vi "migrate files.vi"() -> ()   [LabVIEW 2013]
uses:
  <vilib>/NI/Configuration Framework/class discovery singleton/class discovery singleton methods.ctl
  <vilib>/NI/Configuration Framework/tree serializer/memory hierarchy.ctl
  <vilib>/NI/Configuration Framework/tree serializer/full hierarchy.ctl
  <vilib>/NI/Configuration Framework/tree serializer/hierarchy element.ctl
  <vilib>/NI/Configuration Framework/serializable configuration/NISE_CEF_serializable configuration.lvclass
  <vilib>/NI/Tag Bus Data Framework/Configuration Editor/Classes/Systems/Systems.lvclass
  <vilib>/NI/Configuration Framework/serializable configuration/NISE_CEF_serializable configuration.lvclass/NISE_CEF_serializable configuration.ctl
  <vilib>/NI/Tag Bus Data Framework/core targets/cRIO/PLTarget cRIO.lvclass
  <vilib>/NI/Tag Bus Data Framework/core targets/PC/PLTarget PC.lvclass
  <vilib>/NI/TBM Engines/Standard Engine/Editor Node/Standard Engine Editor Node.lvclass
  <vilib>/NI/Configuration Framework/serializable node/NISE_CEF_serializable node.lvclass
  <vilib>/NI/Tag Bus Data Framework/Framework Configuration Classes/platypus configuration/PLConfigurationSerializer.lvlib
  <vilib>/NI/Configuration Framework/class discovery singleton/class discovery singleton.lvlib
  <vilib>/NI/Configuration Framework/tree serializer/NISE_CEF_TreeSerializer.lvlib
panel:
  out "created paths":path[](array[path])
  in  "cRIO (F=PC)":bool=TRUE
  in  "Path":path
  in  "Plugin Search Paths":path[](array[path])=[path "C:/Program Files (x86)/National Instruments/LabVIEW 2013/vi.lib/NI/Tag Bus Data Framework", path "C:/Program Files (x86)/National Instruments/LabVIEW 2013/vi.lib/NI/TBM Engines", path "C:/Program Files (x86)/National Instruments/LabVIEW 2013/vi.lib/NI/TBM Modules"]
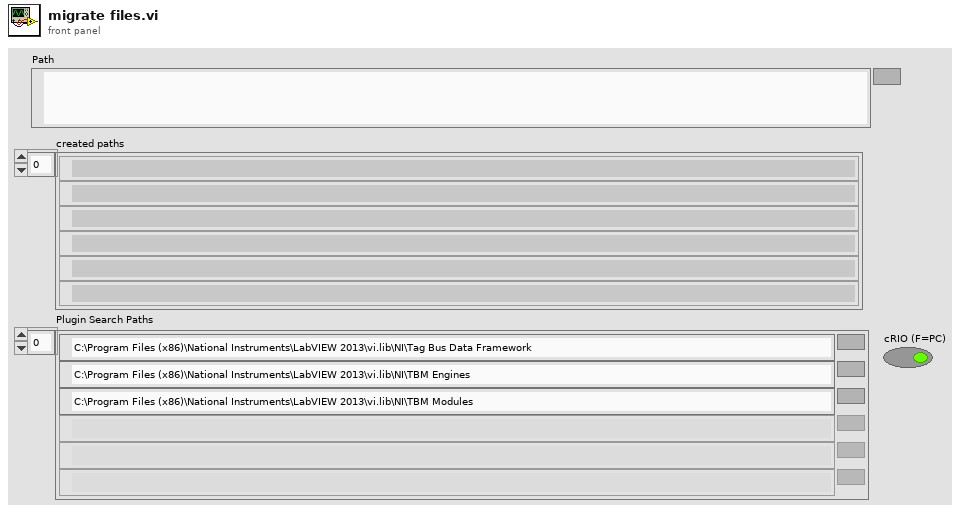
[diagram p1: front panel]
types:
  T1 = typedef "class discovery singleton.lvlib/class discovery singleton methods.ctl" = enum16{"add search paths", "load class by name", "list available classes", "get class path"}
  T2 = typedef "NISE_CEF_TreeSerializer.lvlib/memory hierarchy.ctl" = cluster{"hierarchy structure":T3, "instance data":refnum<class "NISE_CEF_serializable configuration.lvclass">[]}
  T3 = typedef "NISE_CEF_TreeSerializer.lvlib/full hierarchy.ctl" = cluster{"root":string, "hierarchy":T4[]}
  T4 = typedef "NISE_CEF_TreeSerializer.lvlib/hierarchy element.ctl" = cluster{"current node":string, "children":string[]}
  T5 = typedef "PLConfigurationSerializer.lvlib/systems cluster.ctl" = cluster{"System Configuration":refnum<class "PL_System Configuration.lvclass">, "targets":T6[]}
  T6 = typedef "PLConfigurationSerializer.lvlib/targets cluster.ctl" = cluster{"Target Configuration":refnum<class "PL_Target Configuration.lvclass">, "engines":T7[]}
  T7 = typedef "PLConfigurationSerializer.lvlib/engines cluster.ctl" = cluster{"engine configuration":refnum<class "engine configuration.lvclass">, "modules":refnum<class "TBM module configuration.lvclass">[]}
  T8 = typedef "NISE_CEF_TreeSerializer.lvlib/flat hierarchy.ctl" = cluster{"hierarchy structure":T3, "instance data":T9[]}
  T9 = typedef "NISE_CEF_TreeSerializer.lvlib/instance data.ctl" = cluster{"ID":string, "Alias":string, "class":string, "version":string, "data":string}
  T10 = typedef "NISE_CEF_TreeSerializer.lvlib/base file format.ctl" = cluster{"version":string, "data":string}
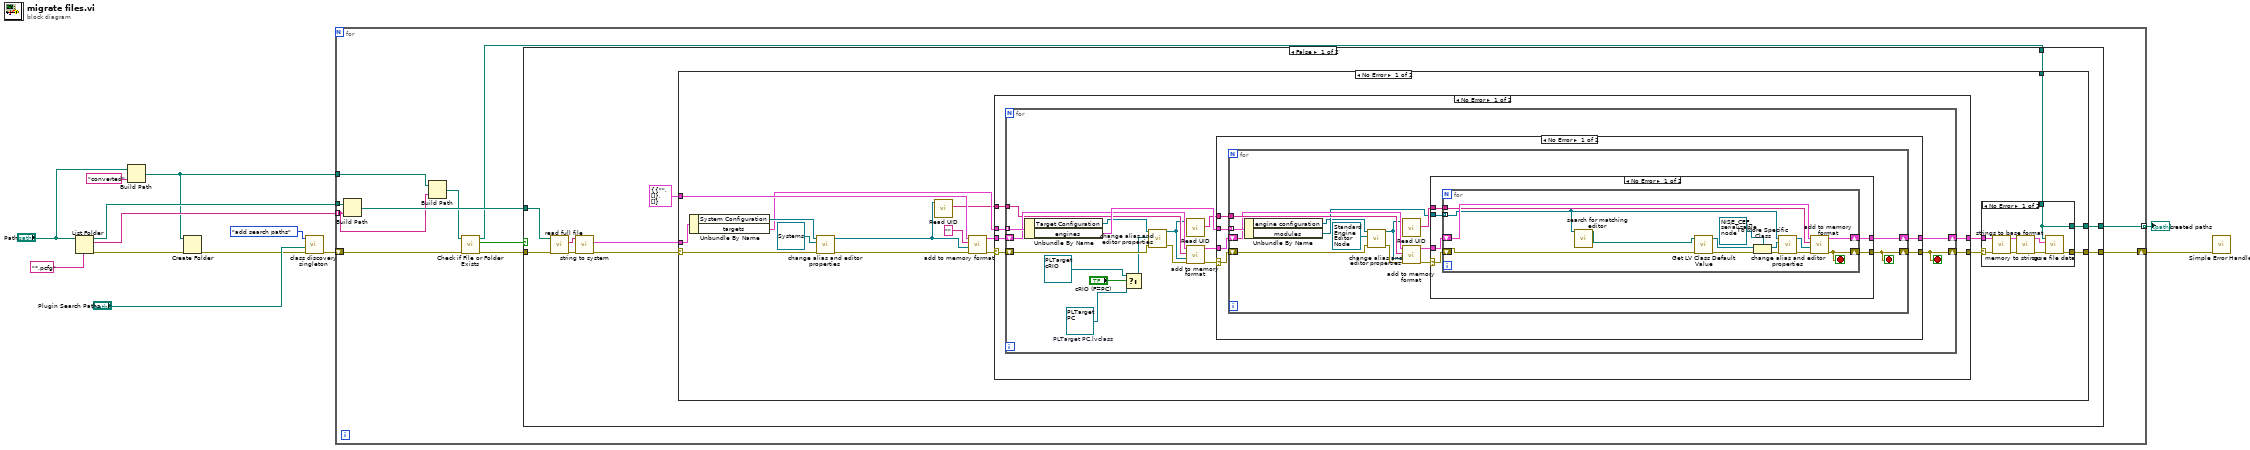
[diagram p0: block diagram]
diagram:
  n1 = List Folder(path="Path", pattern="*.pcfg") -> (path out=w7:path, filenames=w6:string[], error out=w9:errorcluster)  [unwired: 2 in, 1 out]
  n2 = Build Path(base path="Path", name or relative path="converted") -> (appended path=w2:path)
  n3 = Create Folder(path (use dialog)=w2, error in=w9) -> (error out=w5:errorcluster)  [unwired: 1 in, 2 out]
  n4 = call <vilib>:"class discovery singleton.vi"("error in"=w5, "Plugin Search Paths"="Plugin Search Paths", "method"=class_discovery_singleton_methods."add search paths") -> ("error out"=w8:errorcluster)  [unwired: 5 in, 3 out]
  n5 = for {
    shift-right: [w24] -> w11
    shift-left: w8 -> [w23]
    tunnel: w7 -> [w21]
    tunnel: w6 -> [w20] mode=indexing
    tunnel: w2 -> [w17]
    tunnel: [w14] -> w1 mode=indexing
    n6 = Build Path(base path=w21, name or relative path=w20) -> (appended path=w22:path)
    n7 = Build Path(base path=w17, name or relative path=w20) -> (appended path=w18:path)
    n8 = call <vilib>:"Check if File or Folder Exists.vi"("error in (no error)"=w23, "path"=w18) -> ("error out"=w19:errorcluster, "file or folder exists?"=w16:bool, "dup path"=w15:path)  [unwired: 7 in]
    n9 = case shown="False" w16 {
      tunnel: [w31 w131] -> w24
      tunnel: w19 -> [w28 w131]
      tunnel: w22 -> [w27 _]
      tunnel: w15 -> [w26 _]
      tunnel: [w25 _] -> w14
      frame False {
        n10 = call <vilib>:"read full file.vi"("error in"=w28, "file path"=w27) -> ("error out"=w34:errorcluster, "data"=w33:string)  [unwired: 8 in]
        n11 = call <vilib>:"string to system.vi"("error in"=w34, "data"=w33) -> ("error out"=w32:errorcluster, "system"=w30:T5)  [unwired: 8 in]
        n12 = case shown="No Error" w32 {
          selector: w32 -> [w46 w130]
          tunnel: [w39 w130] -> w31
          tunnel: w30 -> [w51 _]
          tunnel: T2 {"hierarchy structure"={"root"="", "hierarchy"=[]}, "instance data"=[]} ("memory hierarchy in") -> [w47 _]
          tunnel: w26 -> [w36 _]
          tunnel: [w35 _] -> w25
          frame No Error {
            n13 = Unbundle By Name(w51) -> ("System Configuration"=w49:refnum<class "PL_System Configuration.lvclass">, "targets"=w44:T6[])
            n14 = call "change alias and editor properties.vi"("error in"=w46, "default node"=refnum<class "Systems.lvclass"> refnum ("Tag Editor Core:Systems.lvclass"), "PL_System Configuration in"=w49) -> ("error out"=w48:errorcluster, "PL_System Configuration out"=w43:refnum<class "PL_System Configuration.lvclass">)  [unwired: 7 in]
            n15 = call <vilib>:"Read UID.vi"("configuration in"=w43) -> ("instance id"=w42:string)  [unwired: 8 in, 2 out]
            n16 = call <vilib>:"add to memory format.vi"("error in"=w48, "NISE_CEF_serializable configuration in"=w43, "parent ID"="", "memory hierarchy in"=w47) -> ("error out"=w41:errorcluster, "memory hierarchy out"=w45:T2)  [unwired: 6 in]
            n17 = case shown="No Error" w41 {
              selector: w41 -> [w62 w129]
              tunnel: w45 -> [w66 w128]
              tunnel: w44 -> [w65 _]
              tunnel: [w64 w129] -> w40
              tunnel: w42 -> [w63 _]
              tunnel: [w61 w128] -> w38
              frame No Error {
                n18 = for {
                  shift-right: [w82] -> w64
                  shift-left: w62 -> [w79]
                  shift-right: [w75] -> w61
                  shift-left: w66 -> [w80]
                  tunnel: w65 -> [w83] mode=indexing
                  tunnel: w63 -> [w78]
                  stop <- w82 stop-if-true
                  w70 = refnum<class "PLTarget PC.lvclass"> refnum  # PLTarget PC.lvclass
                  n19 = Unbundle By Name(w83) -> ("Target Configuration"=w72:refnum<class "PL_Target Configuration.lvclass">, "engines"=w81:T7[])
                  n20 = Select(t=refnum<class "PLTarget cRIO.lvclass"> refnum ("PLTarget cRIO.lvclass"), s="cRIO (F=PC)", f=w70) -> (s? t:f=w67:refnum<class "Targets.lvclass">)
                  n21 = call "change alias and editor properties.vi"("error in"=w79, "default node"=w67, "PL_System Configuration in"=w72) -> ("error out"=w74:errorcluster, "PL_System Configuration out"=w73:refnum<class "PL_Target Configuration.lvclass">)  [unwired: 7 in]
                  n22 = call <vilib>:"Read UID.vi"("configuration in"=w73) -> ("instance id"=w77:string)  [unwired: 8 in, 2 out]
                  n23 = call <vilib>:"add to memory format.vi"("error in"=w74, "NISE_CEF_serializable configuration in"=w73, "parent ID"=w78, "memory hierarchy in"=w80) -> ("error out"=w71:errorcluster, "memory hierarchy out"=w76:T2)  [unwired: 6 in]
                  n24 = case shown="No Error" w71 {
                    selector: w71 -> [w84 w126]
                    tunnel: [w89 w126] -> w82
                    tunnel: w81 -> [w88 _]
                    tunnel: w77 -> [w87 _]
                    tunnel: w76 -> [w86 w127]
                    tunnel: [w85 w127] -> w75
                    frame No Error {
                      n25 = for {
                        shift-right: [w102] -> w89
                        shift-left: w84 -> [w101]
                        tunnel: w88 -> [w103] mode=indexing
                        tunnel: w87 -> [w100]
                        shift-right: [w95] -> w85
                        shift-left: w86 -> [w98]
                        stop <- w102 stop-if-true
                        n26 = Unbundle By Name(w103) -> ("engine configuration"=w92:refnum<class "engine configuration.lvclass">, "modules"=w94:refnum<class "TBM module configuration.lvclass">[])
                        n27 = call "change alias and editor properties.vi"("error in"=w101, "default node"=refnum<class "Standard Engine Editor Node.lvclass"> refnum ("Standard Engine Editor Node.lvclass"), "PL_System Configuration in"=w92) -> ("error out"=w93:errorcluster, "PL_System Configuration out"=w91:refnum<class "engine configuration.lvclass">)  [unwired: 7 in]
                        n28 = call <vilib>:"Read UID.vi"("configuration in"=w91) -> ("instance id"=w99:string)  [unwired: 8 in, 2 out]
                        n29 = call <vilib>:"add to memory format.vi"("error in"=w93, "NISE_CEF_serializable configuration in"=w91, "parent ID"=w100, "memory hierarchy in"=w98) -> ("error out"=w97:errorcluster, "memory hierarchy out"=w96:T2)  [unwired: 6 in]
                        n30 = case shown="No Error" w97 {
                          selector: w97 -> [w107 w125]
                          tunnel: [w109 w125] -> w102
                          tunnel: w99 -> [w108 _]
                          tunnel: w96 -> [w106 w124]
                          tunnel: [w105 w124] -> w95
                          tunnel: w94 -> [w104 _]
                          frame No Error {
                            n31 = for {
                              shift-right: [w118] -> w109
                              shift-left: w107 -> [w110]
                              tunnel: w108 -> [w121]
                              shift-right: [w122] -> w105
                              shift-left: w106 -> [w123]
                              tunnel: w104 -> [w112] mode=indexing
                              stop <- w118 stop-if-true
                              n32 = call "search for matching editor.vi"("LabVIEW Object in"=w112) -> ("appended path"=w111:path)  [unwired: 10 in]
                              n33 = call <vilib>:"Get LV Class Default Value.vi"("error in (no error)"=w110, "class path"=w111) -> ("error out"=w117:errorcluster, "object"=w115:refnum<class>)  [unwired: 8 in]
                              n34 = To More Specific Class(target class=refnum<class "NISE_CEF_serializable node.lvclass"> refnum ("default node"), reference=w115, error in=w117) -> (specific class reference=w113:refnum<class "NISE_CEF_serializable node.lvclass">, error out=w116:errorcluster)
                              n35 = call "change alias and editor properties.vi"("error in"=w116, "default node"=w113, "PL_System Configuration in"=w112) -> ("error out"=w120:errorcluster, "PL_System Configuration out"=w119:refnum<class "TBM module configuration.lvclass">)  [unwired: 7 in]
                              n36 = call <vilib>:"add to memory format.vi"("error in"=w120, "NISE_CEF_serializable configuration in"=w119, "parent ID"=w121, "memory hierarchy in"=w123) -> ("error out"=w118:errorcluster, "memory hierarchy out"=w122:T2)  [unwired: 6 in]
                            }
                          }
                          frame Error {
                          }
                        }
                      }
                    }
                    frame Error {
                    }
                  }
                }
              }
              frame Error {
              }
            }
            n37 = case shown="No Error" w40 {
              selector: w40 -> [w59 w60]
              tunnel: [w53 w60] -> w39
              tunnel: w38 -> [w58 _]
              tunnel: w36 -> [w52 _]
              tunnel: [w52 _] -> w35
              frame No Error {
                n38 = call <vilib>:"memory to strings.vi"("error in"=w59, "memory hierarchy"=w58) -> ("error out"=w57:errorcluster, "1.0.0"=w56:T8)  [unwired: 8 in]
                n39 = call <vilib>:"strings to base format.vi"("error in"=w57, "1.0.0"=w56) -> ("error out"=w54:errorcluster, "format"=w55:T10)  [unwired: 8 in]
                n40 = call <vilib>:"save file data.vi"("error in"=w54, "format"=w55, "Path"=w52) -> ("error out"=w53:errorcluster)  [unwired: 8 in]
              }
              frame Error {
              }
            }
          }
          frame Error {
          }
        }
      }
      frame True {
      }
    }
  }
  "created paths" <- w1
  n41 = call <vilib>:"Simple Error Handler.vi"("error in (no error)"=w11) -> ()  [unwired: 4 in, 5 out]
